vi "Stop Acquisition.vi"(8 "error in (no error)":errorcluster, 11 "Hardware Resources in":T1) -> (0 "error out":errorcluster)   [LabVIEW 2014, in "Acquisition.lvlib"]
doc: "Stops the acquisition."
uses:
  Acquisition.lvlib
  Hardware Configuration.ctl
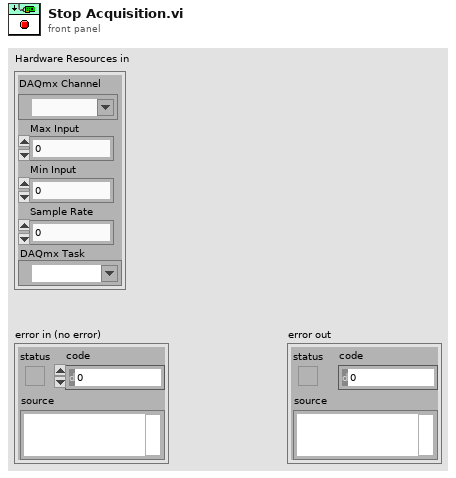
[diagram p1: front panel]
types:
  T1 = typedef "Acquisition.lvlib/Hardware Configuration.ctl" = cluster{"DAQmx Channel":tag, "Max Input":dbl, "Min Input":dbl, "Sample Rate":dbl, "DAQmx Task":refnum<k21>}
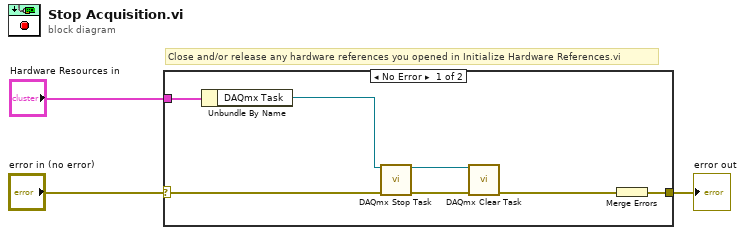
[diagram p0: block diagram]
diagram:
  # "Close and/or release any hardware references you opened in Initialize Hardware References.vi"
  n1 = case shown="No Error" "error in (no error)" {
    selector: "error in (no error)" -> [w8 w11]
    tunnel: [w10 w11] -> w2
    tunnel: "Hardware Resources in" -> [w9 _]
    frame No Error {
      n2 = Unbundle By Name(w9) -> ("DAQmx Task"=w7:refnum<k21>)
      n3 = call <vilib>:"DAQmx Stop Task.vi"("task/channels in"=w7, "error in"=w8) -> ("task out"=w6:refnum<k21>, "error out"=w5:errorcluster)  [unwired: 12 in]
      n4 = call <vilib>:"DAQmx Clear Task.vi"("task in"=w6, "error in"=w5) -> ("error out"=w4:errorcluster)  [unwired: 13 in]
      n5 = Merge Errors(w4) -> (w10:errorcluster)
    }
    frame Error {
    }
  }
  "error out" <- w2
